vi "CIC FXPi18x1.vi"(0 "input":fxp<+/-,18,1>, 1 "reset":bool, 5 "decimation factor":fxp<+,16,16>, 7 "config valid":bool, 9 "input valid":bool) -> (4 "output":fxp<+,64,64>, 10 "output valid":bool)   [LabVIEW 2017, in "Lock-In Amplifier Example FPGA.lvlib"]
uses:
  Lock-In Amplifier Example FPGA.lvlib
  <vilib>/rvi/IPIntegrationNode/IPINode_Typedef/niFpgaIPINodeSupportedFamilies.ctl
  <vilib>/rvi/IPIntegrationNode/IPINode_Utilities/niFpgaIPINodeSimCore.vi
  <vilib>/rvi/XilinxIP/XIPIN_XNode/niFpgaXIPIN.xnode
  CIC FXPi18x1/CIC Compiler/xsim.dir/CIC_Compiler_46A5B37C04AB4F31B6372087A31BC6A8/xsimk_46A5B37C04AB4F31B6372087A31BC6A8.dll
  <vilib>/rvi/IPIntegrationNode/IPINode_Xnode/niFpgaIPINode.xnode
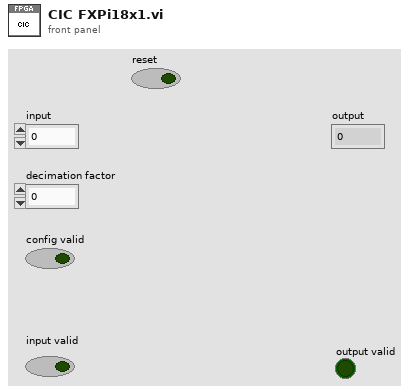
[diagram p1: front panel]
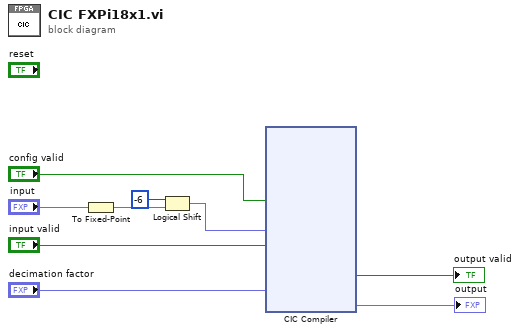
[diagram p0: block diagram]
diagram:
  n1 = To Fixed-Point(number="input") -> (fixed-point=w8:fxp<+/-,24,1>)  [unwired: 1 in]
  n2 = Logical Shift(y=i16 -6, x=w8) -> (x << y=w5:fxp<+/-,24,1>)
  n3 = xnode ("CIC Compiler")("s_axis_config_tvalid"="config valid", "s_axis_data_tdata"=w5, "s_axis_data_tvalid"="input valid", "s_axis_config_tdata"="decimation factor") -> ("m_axis_data_tvalid"=→"output valid":bool, "m_axis_data_tdata"=→"output":fxp<+,64,64>)  [unwired: 2 out]
